vi "VD-convert_for_graph.vi"(10 "VNA data":T1) -> (2 "Graph Data":T2)   [LabVIEW 2020, in "VD-LV-LiteVNA.lvclass"]
uses:
  VD-LV-LiteVNA.lvclass
  VD-graph_data.ctl
  VD-VNA_data.ctl
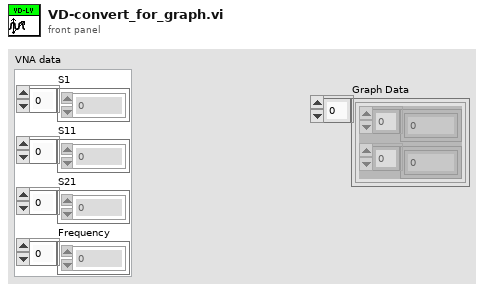
[diagram p1: front panel]
types:
  T1 = typedef "VD-LV-LiteVNA.lvclass/VD-VNA_data.ctl" = cluster{"S1":cdb[], "S11":cdb[], "S21":cdb[], "Frequency":u64[]}
  T2 = typedef "VD-LV-LiteVNA.lvclass/VD-graph_data.ctl" = cluster{u64[], dbl[]}[]
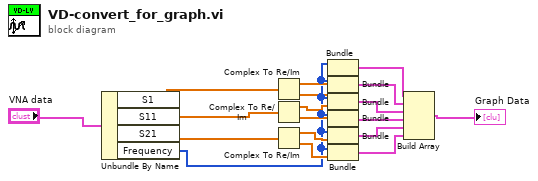
[diagram p0: block diagram]
diagram:
  n1 = Unbundle By Name("VNA data") -> ("S1"=w6:cdb[], "S11"=w5:cdb[], "S21"=w4:cdb[], "Frequency"=w3:u64[])
  n2 = Complex To Re/Im(x + iy=w6) -> (x=w12:dbl[], y=w11:dbl[])
  n3 = Complex To Re/Im(x + iy=w5) -> (x=w10:dbl[], y=w9:dbl[])
  n4 = Complex To Re/Im(x + iy=w4) -> (x=w8:dbl[], y=w7:dbl[])
  n5 = Bundle("Frequency"=w3, w12) -> (w13:cluster{"Frequency":u64[], dbl[]})  [unwired: 1 in]
  n6 = Bundle("Frequency"=w3, w11) -> (w14:cluster{"Frequency":u64[], dbl[]})  [unwired: 1 in]
  n7 = Bundle("Frequency"=w3, w10) -> (w17:cluster{"Frequency":u64[], dbl[]})  [unwired: 1 in]
  n8 = Bundle("Frequency"=w3, w9) -> (w18:cluster{"Frequency":u64[], dbl[]})  [unwired: 1 in]
  n9 = Bundle("Frequency"=w3, w8) -> (w16:cluster{"Frequency":u64[], dbl[]})  [unwired: 1 in]
  n10 = Bundle("Frequency"=w3, w7) -> (w15:cluster{"Frequency":u64[], dbl[]})  [unwired: 1 in]
  n11 = Build Array(w13, w14, w17, w18, w16, w15) -> (→"Graph Data":cluster{"Frequency":u64[], dbl[]}[])
